vi "euler2q.vi"(1 "Eta":dbl[](array[numeric])) -> (0 "q":dbl[](array[numeric]))   [LabVIEW 2014]
uses:
  <vilib>/imath/engines/lvmath2/RunTimeEngine/Managers/WorkSpace/UID Generator.vi
  <vilib>/imath/engines/lvmath2/RunTimeEngine/IndexRead/NIMS M(S,S).vi
  <instcachedir>/0/NIMS M(S,S)_AC51E74150A542F7991B9634C66F3096.lvgen/NIMS M(S,S)_AC51E74150A542F7991B9634C66F3096_000.vi
  <vilib>/imathl/engines/lvmath/Functions/Error Handling/Create Error.vi
  <vilib>/imath/engines/lvmath2/RunTimeEngine/BuiltInFunctions/trace/NIMS_trace.vi
  <instcachedir>/0/NIMS_trace_D2062D2237D14A159AD794D274BA148D.lvgen/NIMS_trace_D2062D2237D14A159AD794D274BA148D_000.vi
  <vilib>/imath/engines/lvmath2/RunTimeEngine/RunTimeType/NIMS_RunTimeType_From StrictType (excl LVString).vi
  <instcachedir>/0/NIMS_RunTimeType_From StrictType (excl LVString)_15A5391EEA9C4AACB9955AC755B83D29.lvgen/NIMS_RunTimeType_From StrictType (excl LVString)_15A5391EEA9C4AACB9955AC755B83D29_000.vi
  <vilib>/imath/engines/lvmath2/RunTimeEngine/ErrorHandling/NIMS_Error From Error Code.vi
  <vilib>/imath/engines/lvmath2/RunTimeEngine/LocalVariableDefStatement/MC_LocalVariableDefStatement_Display.vi
  <vilib>/imath/engines/lvmath2/RunTimeEngine/BuiltInFunctions/max/1 input/NIMS_max(RV).vi
  <instcachedir>/0/NIMS_max(RV)_237633DB1D604D5BA7001287DF3C7957.lvgen/NIMS_max(RV)_237633DB1D604D5BA7001287DF3C7957_000.vi
  <vilib>/imath/engines/lvmath2/RunTimeEngine/IndexRead/NIMS V(S).vi
  <instcachedir>/0/NIMS V(S)_0488751826AF41519A22953C041130DC.lvgen/NIMS V(S)_0488751826AF41519A22953C041130DC_000.vi
  <vilib>/imath/engines/lvmath2/RunTimeEngine/BuiltInFunctions/abs/NIMS_abs(signed).vi
  <instcachedir>/0/NIMS_abs(signed)_C4FCB8E6058B49B797C7C8D53CA5F6EC.lvgen/NIMS_abs(signed)_C4FCB8E6058B49B797C7C8D53CA5F6EC_002.vi
  <vilib>/imath/engines/lvmath2/RunTimeEngine/ErrorHandling/NIMS_Create Error From Enums.vi
  <vilib>/imath/engines/lvmath2/RunTimeEngine/VariableToken/NIMS_VariableToken_CondDefined.vi
  <instcachedir>/0/NIMS_VariableToken_CondDefined_EE8DD211A89249938CE6537267F5C9B3.lvgen/NIMS_VariableToken_CondDefined_EE8DD211A89249938CE6537267F5C9B3_004.vi
  <vilib>/imath/engines/lvmath2/RunTimeEngine/ArithmeticOperatorToken/NIMS_ArithmeticOperator_multmx(RV,CV)-internal.vi
  <instcachedir>/0/NIMS_ArithmeticOperator_multmx(RV,CV)-internal_E181434B092F4BAFA1B7E5F22D537F51.lvgen/NIMS_ArithmeticOperator_multmx(RV,CV)-internal_E181434B092F4BAFA1B7E5F22D537F51_005.vi
  <vilib>/imath/engines/lvmath2/RunTimeEngine/Managers/SymbolTable/Clear UID.vi
  <vilib>/imath/engines/lvmath2/RunTimeEngine/NodeEndStatement/NIMS_NodeEndStatement_Output.vi
  <instcachedir>/0/NIMS_NodeEndStatement_Output_53EC0D466D134D7ABD903AC30B43404B.lvgen/NIMS_NodeEndStatement_Output_53EC0D466D134D7ABD903AC30B43404B_005.vi
  <vilib>/imath/engines/lvmath2/RunTimeEngine/ErrorHandling/NIMS_Finalize Error.vi
  <vilib>/imath/engines/lvmath2/RunTimeEngine/Managers/SymbolTable/NIMS_WorkSpace.lvlib
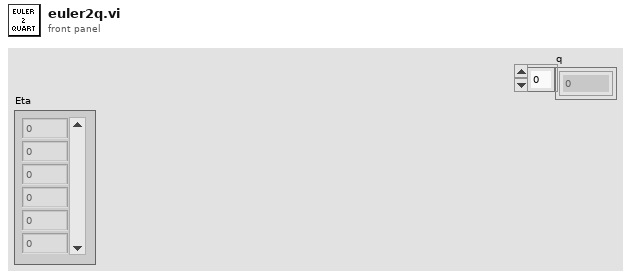
[diagram p1: front panel]
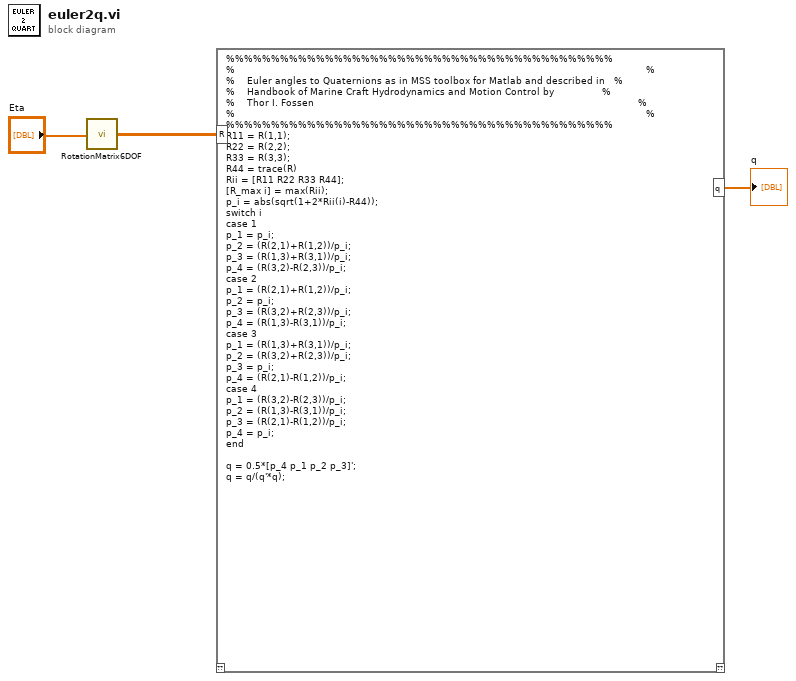
[diagram p0: block diagram]
diagram:
  n1 = call "RotationMatrix6DOF.vi"("Eta"="Eta") -> ("R"=w2:dbl[][])
  n2 = mathscript code="%%%%%%%%%%%%%%%%%%%%%%%%%%%%%%%%%%%%%%%%%%%\n%                                                                                                                                         %\n%    Euler angles to Quaternions as in MSS toolbox for Matlab and described in   %\n%    Handbook of Marine Craft Hydrodynamics and Motion Control by                %\n%    Thor I. Fossen                                                                                                            %\n%                                                                                                                                         %\n%%%%%%%%%%%%%%%%%%%%%%%%%%%%%%%%%%%%%%%%%%%\nR11 = R(1,1);\nR22 = R(2,2);\nR33 = R(3,3);\nR44 = trace(R)\nRii = [R11 R22 R33 R44];\n[R_max i] = max(Rii);\np_i = abs(sqrt(1+2*Rii(i)-R44));\nswitch i\ncase 1\np_1 = p_i;\np_2 = (R(2,1)+R(1,2))/p_i;\np_3 = (R(1,3)+R(3,1))/p_i;\np_4 = (R(3,2)-R(2,3))/p_i;\ncase 2\np_1 = (R(2,1)+R(1,2))/p_i;\np_2 = p_i;\np_3 = (R(3,2)+R(2,3))/p_i;\np_4 = (R(1,3)-R(3,1))/p_i;\ncase 3\np_1 = (R(1,3)+R(3,1))/p_i;\np_2 = (R(3,2)+R(2,3))/p_i;   \np_3 = p_i;\np_4 = (R(2,1)-R(1,2))/p_i;   \ncase 4\np_1 = (R(3,2)-R(2,3))/p_i;\np_2 = (R(1,3)-R(3,1))/p_i;\np_3 = (R(2,1)-R(1,2))/p_i;   \np_4 = p_i;\nend\n\nq = 0.5*[p_4 p_1 p_2 p_3]';\nq = q/(q'*q);"("R"=w2) -> ("q"=→"q":dbl[])  [unwired: 1 in, 1 out]
